vi "2LOOPs Parallelism.vi"() -> ()   [LabVIEW 2019]
panel:
  out "Cmd-indicator":string
  out "ErrO":errorcluster
  in  "ErrI":errorcluster
  in  "Exit":bool
  in  "OK":bool
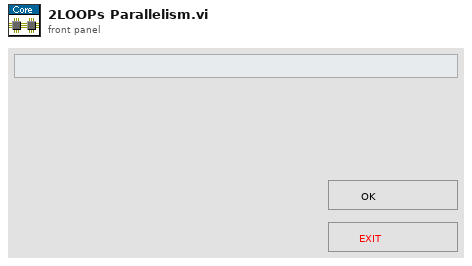
[diagram p1: front panel]
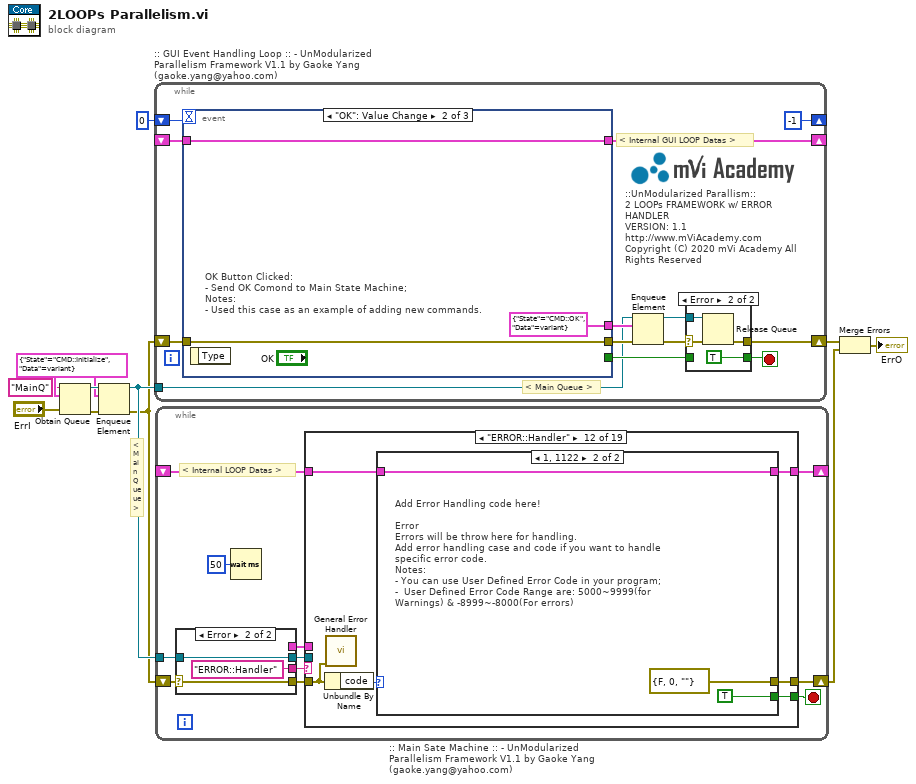
[diagram p0: block diagram]
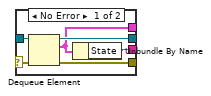
[diagram p2: hidden frame]
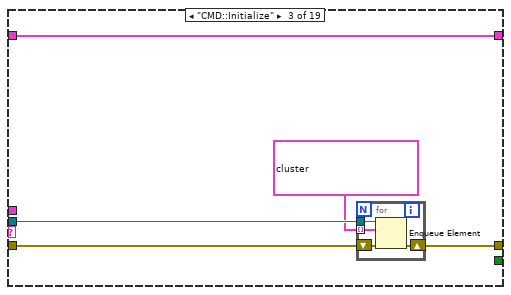
[diagram p5: hidden frame]
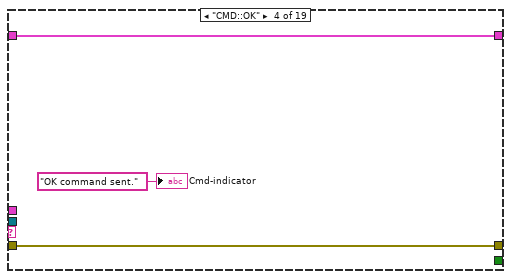
[diagram p6: hidden frame]
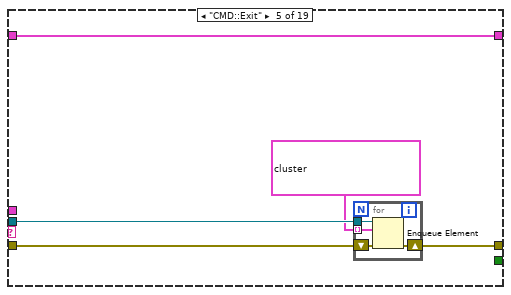
[diagram p7: hidden frame]
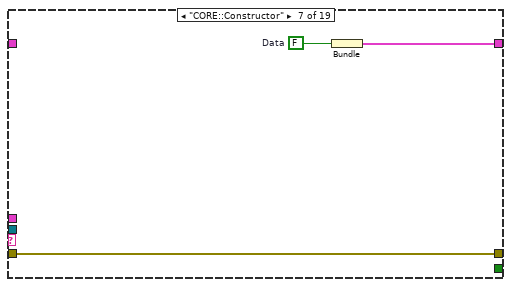
[diagram p9: hidden frame]
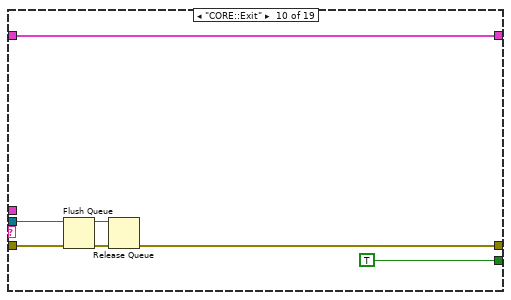
[diagram p12: hidden frame]
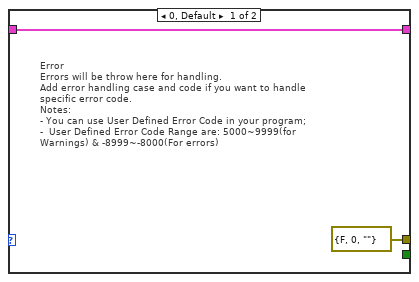
[diagram p14: hidden frame]
diagram:
  w7 = cluster{"State":string, "Data":variant} {"State"="CMD::Initialize", "Data"=variant} ("MainQueue")
  # "< Main Queue >"
  n1 = Obtain Queue(name (unnamed)="MainQ", element data type=w7, error in (no error)="ErrI") -> (queue out=w9:refnum<queue>, error out=w8:errorcluster)  [unwired: 2 in, 1 out]
  n2 = Enqueue Element(queue=w9, element=w7, error in (no error)=w8) -> (queue out=w5:refnum<queue>, error out=w4:errorcluster)  [unwired: 2 out]
  n3 = while ":: GUI Event Handling Loop :: - UnModularized Parallelism Framework V1.1 by Gaoke Yang (gaoke.yang@yahoo.com)" {
    tunnel: w5 -> [w14]
    shift-right: [w23] -> w11
    shift-left: w4 -> [w24]
    shift-right: [-1] -> _
    shift-left: 0 -> [w21]
    shift-right: [w20] -> _
    shift-left: _ -> [w19]
    stop <- w17 stop-if-true
    # "::UnModularized Parallism::\n2 LOOPs FRAMEWORK w/ ERROR HANDLER\nVERSION: 1.1\nhttp://www.mViAcademy.com\nCopyright (C) 2020 mVi Academy All Rights Reserved"
    # "< Internal GUI LOOP Datas >"
    # "< Main Queue >"
    n4 = event shown="[1] \"OK\": Value Change" {
      selector: _ -> [_ _ _]
      dyn-events: _ -> [_ _ _]
      timeout: w21 -> [_ _ _]
      tunnel: [_ _ TRUE ("Exit")] -> w18
      tunnel: w24 -> [w34 w37 w38]
      tunnel: [w34 w37 w38] -> w16
      tunnel: [_ cluster{"State":string, "Data":variant} {"State"="CMD::OK", "Data"=variant} ("Packet") cluster{"State":string, "Data":variant} {"State"="CMD::Exit", "Data"=variant} ("Packet")] -> w15
      tunnel: [w32 w36 w41] -> w20
      tunnel: w19 -> [_ w36 w41]
      event Timeout {
        w33 = FALSE  # GUI Data Example
        # "Timeout:\n- This Case will only bee excuted for 1 time since timeout=0;\nNotes:\n- Used this place as a GUI Initializer."
        n5 = event-data() -> ()  [unwired: 2 out]
        n6 = local write "Cmd-indicator"("" ("Cmd-indicator")) -> ()
        n7 = Bundle("GUI Data Example"=w33) -> (w32:cluster{"GUI Data Example":bool})  [unwired: 1 in]
      }
      event "OK": Value Change {
        # "OK Button Clicked:\n- Send OK Comond to Main State Machine;\nNotes:\n- Used this case as an example of adding new commands."
        n8 = event-data() -> ()  [unwired: 2 out]
      }
      event "Exit": Value Change; Panel Close {
        # "Exit Button clicked or panel was closed\n- Send Exit commands and Exit Application\nNotes:"
        n9 = event-data() -> ()  [unwired: 2 out]
      }
    }
    n10 = Enqueue Element(queue=w14, element=w15, error in (no error)=w16) -> (queue out=w12:refnum<queue>, error out=w13:errorcluster)  [unwired: 2 out]
    n11 = case shown="Error" w13 {
      selector: w13 -> [w26 w29]
      tunnel: [w26 w27] -> w23
      tunnel: w18 -> [w25 _]
      tunnel: [w25 TRUE ("Exit")] -> w17
      tunnel: w12 -> [_ w28]
      frame No Error {
      }
      frame Error {
        n12 = Release Queue(queue=w28, error in (no error)=w29) -> (error out=w27:errorcluster)  [unwired: 1 in, 2 out]
      }
    }
  }
  n13 = while ":: Main Sate Machine :: - UnModularized Parallelism Framework V1.1 by Gaoke Yang (gaoke.yang@yahoo.com)" {
    tunnel: w5 -> [w52]
    shift-right: [w44] -> w3
    shift-left: w4 -> [w43]
    shift-right: [w46] -> _
    shift-left: _ -> [w45]
    stop <- w49 stop-if-true
    # "< Internal LOOP Datas >"
    n14 = case shown="Error" w43 {
      selector: w43 -> [w53 w61]
      tunnel: w52 -> [w58 w59]
      tunnel: [w57 w61] -> w51
      tunnel: [w56 w59] -> w50
      tunnel: [w55 "ERROR::Handler" ("State")] -> w48
      tunnel: [w54 _] -> w47
      frame No Error {
        n15 = Dequeue Element(queue=w58, error in (no error)=w53) -> (queue out=w56:refnum<queue>, element=w54:cluster{"State":string, "Data":variant}, error out=w57:errorcluster)  [unwired: 2 out]
        n16 = Unbundle By Name(w54) -> ("State"=w55:string)
      }
      frame Error {
      }
    }
    n17 = Wait (ms)(milliseconds to wait=u32 50) -> ()  [unwired: 1 out]
    n18 = case shown="\"ERROR::Handler\"" w48 {
      tunnel: [w62 w65 w69 w76 w81 w88 w91 w93 w95 w96 w104 w106 w116 w118 w120 w123 w125 w127 w128] -> w44
      tunnel: [_ _ _ _ _ _ _ _ _ TRUE _ w105 _ _ _ _ _ _ _] -> w49
      tunnel: w50 -> [_ _ w68 _ w79 _ _ _ _ w101 _ _ _ _ _ _ _ _ _]
      tunnel: w51 -> [w62 w65 w67 w76 w80 w88 w91 w93 w95 w100 w104 w109 w116 w118 w120 w123 w125 w127 w128]
      tunnel: w47 -> [_ _ _ _ _ _ _ _ _ _ _ _ _ _ _ _ _ _ _]
      tunnel: [w63 w64 w70 w77 w82 w87 w89 w92 w94 w98 w103 w107 w117 w119 w121 w122 w124 w126 w129] -> w46
      tunnel: w45 -> [w63 w64 w70 w77 w82 w87 _ w92 w94 w98 w103 w108 w117 w119 w121 w122 w124 w126 w129]
      frame "IDLE", Default {
      }
      frame "-------- Commands ---------" {
      }
      frame "CMD::Initialize" {
        n19 = for {
          shift-right: [w73] -> w69
          shift-left: w67 -> [w74]
          tunnel: cluster{"State":string, "Data":variant}[] [{"State"="CORE::Constructor", "Data"=variant}, {"State"="CORE::Initialize", "Data"=variant}] -> [w72] mode=indexing
          tunnel: w68 -> [w71]
          n20 = Enqueue Element(queue=w71, element=w72, error in (no error)=w74) -> (error out=w73:errorcluster)  [unwired: 3 out]
        }
      }
      frame "CMD::OK" {
        "Cmd-indicator" <- "OK command sent." ("Cmd-indicator")
      }
      frame "CMD::Exit" {
        n21 = for {
          shift-right: [w85] -> w81
          shift-left: w80 -> [w86]
          tunnel: w79 -> [w84]
          tunnel: cluster{"State":string, "Data":variant}[] [{"State"="CORE::DeConstructor", "Data"=variant}, {"State"="CORE::Exit", "Data"=variant}] -> [w83] mode=indexing
          n22 = Enqueue Element(queue=w84, element=w83, error in (no error)=w86) -> (error out=w85:errorcluster)  [unwired: 3 out]
        }
      }
      frame "------------ Core ------------" {
      }
      frame "CORE::Constructor" {
        w90 = FALSE  # Data
        n23 = Bundle("Data"=w90) -> (w89:cluster{"Data":bool})  [unwired: 1 in]
      }
      frame "CORE::Initialize" {
      }
      frame "CORE::DeConstructor" {
      }
      frame "CORE::Exit" {
        n24 = Flush Queue(queue=w101, error in (no error)=w100) -> (queue out=w97:refnum<queue>, error out=w99:errorcluster)  [unwired: 1 out]
        n25 = Release Queue(queue=w97, error in (no error)=w99) -> (error out=w96:errorcluster)  [unwired: 1 in, 2 out]
      }
      frame "----------- Error ------------" {
      }
      frame "ERROR::Handler" {
        n26 = Unbundle By Name(w109) -> ("code"=w110:i32)
        n27 = call <vilib>:"General Error Handler.vi"("error in (no error)"=w109) -> ()  [unwired: 10 in, 5 out]
        n28 = case shown="1, 1122" w110 {
          tunnel: [w112 w115] -> w107
          tunnel: w108 -> [w112 w115]
          tunnel: [errorcluster {"status"=FALSE, "code"=0, "source"=""} ("error out") errorcluster {"status"=FALSE, "code"=0, "source"=""} ("error out")] -> w106
          tunnel: [_ TRUE] -> w105
          frame 0, Default {
            # "Error\nErrors will be throw here for handling.\nAdd error handling case and code if you want to handle specific error code.\nNotes:\n- You can use User Defined Error Code in your program;\n-  User Defined Error Code Range are: 5000~9999(for Warnings) & -8999~-8000(For errors)"
          }
          frame 1, 1122 {
            # "Add Error Handling code here!\n\nError\nErrors will be throw here for handling.\nAdd error handling case and code if you want to handle specific error code.\nNotes:\n- You can use User Defined Error Code in your program;\n-  User Defined Error Code Range are: 5000~9999(for Warnings) & -8999~-8000(For errors)"
          }
        }
      }
      frame "------------  GUI  -------------" {
      }
      frame "GUI::Initialize" {
      }
      frame "GUI::SetCusor" {
      }
      frame "GUI::SetMenu" {
      }
      frame "----------- USER -----------" {
      }
      frame "USER::Case1" {
      }
      frame "USER::Case2" {
      }
    }
  }
  n29 = Merge Errors(w11, w3) -> (→"ErrO":errorcluster)
